vi "Zero Phase Filter (obs, DBL).vi"(7 "init/cont (init:F)":bool, 9 "Forward Coefficients":dbl[](array[numeric]), 10 "Reverse Coefficients":dbl[](array[numeric]), 11 "X":dbl[](array[numeric])) -> (0 "error":i32, 3 "Filtered X":dbl[](array[numeric]))   [LabVIEW 2017, in "NI_AALBase.lvlib"]
doc: "Applies a zero phase filter to an input sequence <B>X</B>. Wire data to the <B>X</B> input to determine the polymorphic instance to use or manually select the instance."
uses:
  <vilib>/Analysis/NI_AALBase.lvlib
  <resource>/lvanlys.dll
panel:
  # "This VI is obsolete !!!\nYou should replace this VI in your diagram with the Zero Phase Filter VI.\n\nNOTE: If you have wired to the init input of this obsolete VI, please be\n            aware that the new Zero Phase Filter VI does not have such input.\n            Because of the non-causal property of zero phase filter, you should\n            use Zero Phase Filter VI in single-shot mode, not continuous mode."
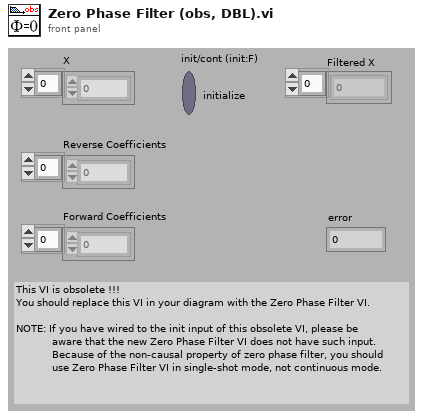
[diagram p1: front panel]
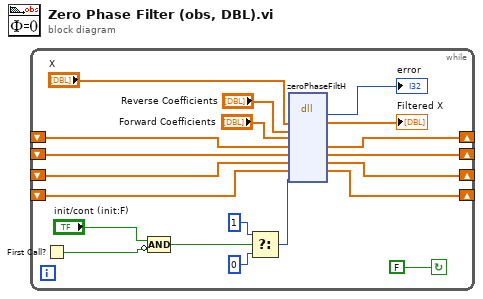
[diagram p0: block diagram]
diagram:
  n1 = while {
    shift-left: _ -> [w13]
    shift-right: [w14] -> _
    shift-left: _ -> [w15]
    shift-right: [w16] -> _
    shift-right: [w12] -> _
    shift-left: _ -> [w11]
    shift-right: [w10] -> _
    shift-left: _ -> [w9]
    stop <- FALSE continue-if-true
    n2 = First Call?() -> (First Call?: T/F=w3:bool)
    n3 = Compound Arithmetic op=AND("init/cont (init:F)", invert w3) -> (w1:bool)
    n4 = Select(t=1, s=w1, f=0) -> (s? t:f=w6:i32)
    n5 = dll-call lib="e:/builds/penguin/labview/branches/2017/dev/dist/resource/lvanlys.*" fn="zeroPhaseFiltH"("X"="X", "Reverse Coefficients"="Reverse Coefficients", "Forward Coefficients"="Forward Coefficients", "x1H"=w15, "x2H"=w13, "y1H"=w11, "y2H"=w9, "reset"=w6) -> (→"error":i32, "X"=→"Filtered X":dbl[], "x1H"=w16:dbl[], "x2H"=w14:dbl[], "y1H"=w12:dbl[], "y2H"=w10:dbl[])  [unwired: 6 in, 2 out]
  }
